vi "set_FTPSettings.vi"(0 "Host_Reference":refnum<class "HGF_Reference.lvclass">, 2 "timeout in ms (-1)":i32=-1, 5 "error in (no error)":errorcluster) -> (14 "dup Host_Reference":refnum<class "HGF_Reference.lvclass">, 19 "error out":errorcluster)   [LabVIEW 2009, in "MoAgSy.lvlib" / "MoAgSy_Host.lvclass"]
doc: "<B>public</B> VI changes FTP Settings of the referenced Host.\nFTP settings are needed to download unknown class code dynamically.\n<B>VI frontpanel has to be shown at vi call.</B>\n\nF.Berck@gsi.de\nGSI Darmstadt 2009"
uses:
  MoAgSy_Host.lvclass
  HGF_BaseClasses/HGF_Reference/HGF_Reference.lvclass
panel:
  in  "FTP Settings":T1={"FTP Host"="", "FTP Username"="", "FTP Password"="", "remote port (21)"=21, "Load new libs from FTP server"=TRUE}
  in  "Cancel":bool
  in  "Apply":bool
  # "Change FTP Settings"
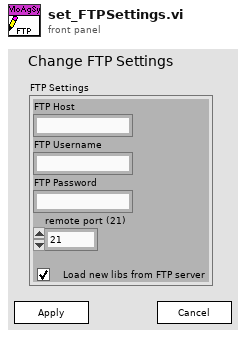
[diagram p1: front panel]
types:
  T1 = cluster{"FTP Host":string, "FTP Username":string, "FTP Password":string, "remote port (21)":u16, "Load new libs from FTP server":bool}
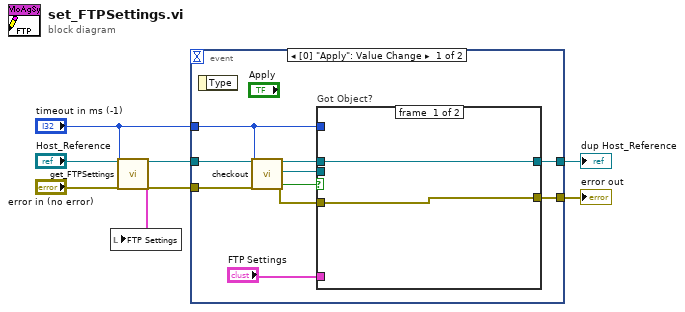
[diagram p0: block diagram]
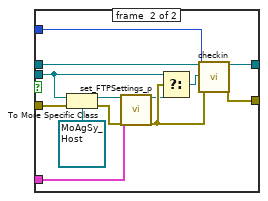
[diagram p2: hidden frame]
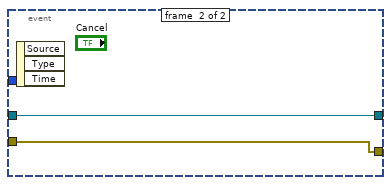
[diagram p3: hidden frame]
diagram:
  n1 = call "get_FTPSettings.vi"("Host_Reference"="Host_Reference", "timeout in ms (-1)"="timeout in ms (-1)", "error in (no error)"="error in (no error)") -> ("dup Host_Reference"=w4:refnum<class "HGF_Reference.lvclass">, "FTP Settings"=w1:T1, "error out"=w2:errorcluster)  [unwired: 14 out]
  n2 = local write "FTP Settings"(w1) -> ()
  n3 = event shown="[0] \"Apply\": Value Change" {
    selector: _ -> [_ _]
    dyn-events: _ -> [_ _]
    timeout: _ -> [_ _]
    tunnel: [w18 w34] -> w8
    tunnel: [w17 w35] -> w7
    tunnel: "timeout in ms (-1)" -> [w13 _]
    tunnel: w4 -> [w12 w35]
    tunnel: w2 -> [w11 w34]
    event #0 {
      n4 = event-data() -> ()  [unwired: 2 out]
      n5 = call "checkout.vi"("HGF_Reference"=w12, "timeout in ms (-1)"=w13, "error in (no error)"=w11) -> ("dup HGF_Reference"=w16:refnum<class "HGF_Reference.lvclass">, "Object"=w14:refnum<class>, "got object?"=w15:bool, "error out"=w10:errorcluster)  [unwired: 13 out]
      n6 = case "Got Object?" shown="True" w15 {
        tunnel: w14 -> [_ w24]
        tunnel: w16 -> [w20 w31]
        tunnel: [w20 w30] -> w17
        tunnel: w13 -> [_ w29]
        tunnel: [w19 w28] -> w18
        tunnel: "FTP Settings" -> [_ w26]
        tunnel: w10 -> [w19 w25]
        frame #0 {
        }
        frame #1 {
          n7 = To More Specific Class(target class=refnum<class "MoAgSy_Host.lvclass"> refnum ("MoAgSy.lvlib:MoAgSy_Host.lvclass"), reference=w24, error in=w25) -> (specific class reference=w27:refnum<class "MoAgSy_Host.lvclass">, error out=w33:errorcluster)
          n8 = call "set_FTPSettings_p.vi"("MoAgSy_Host"=w27, "FTP Settings"=w26, "error in (no error)"=w33) -> ("dup MoAgSy_Host"=w22:refnum<class "MoAgSy_Host.lvclass">, "error out"=w23:errorcluster)  [unwired: 15 out]
          n9 = Select(t=w24, s=w23, f=w22) -> (s? t:f=w21:refnum<class>)
          n10 = call "checkin.vi"("HGF_Reference"=w31, "Object"=w21, "timeout /ms (-1)"=w29, "error in (no error)"=w23) -> ("dup HGF_Reference"=w30:refnum<class "HGF_Reference.lvclass">, "error out"=w28:errorcluster)  [unwired: 14 out]
        }
      }
    }
    event #1 {
      n11 = event-data() -> ()  [unwired: 4 out]
    }
  }
  "dup Host_Reference" <- w7
  "error out" <- w8
